vi "FCI Lip gap.vi"(8 "error in (no error)":errorcluster, 11 "Image 2":T1) -> (0 "error IO":errorcluster, 2 "Lip Gap":sgl format="%.2f")   [LabVIEW 2019, in "Algorithm.lvclass"]
uses:
  FrameworkOverrides/Algorithm.lvclass
  <vilib>/vision/NI_Vision_Development_Module.lvlib
  <vilib>/vision/Measure.llb/Straight Edge Process.ctl
  <vilib>/vision/Measure.llb/Straight Edge Options.ctl
  <vilib>/vision/Measure.llb/Edge Polarity.ctl
  <vilib>/vision/Measure.llb/Edge Options.ctl
  <vilib>/vision/Image Controls.llb/IMAQ Image.ctl
panel:
  out "Image":T1(plugin-control)
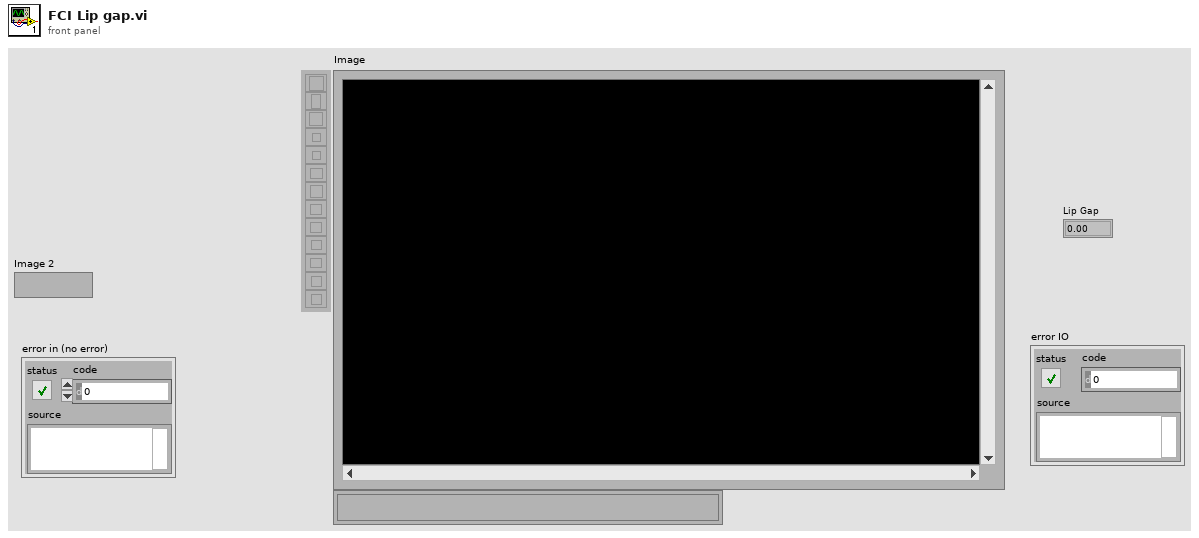
[diagram p1: front panel]
types:
  T1 = typedef "IMAQ Image.ctl" = refnum<image>
  T2 = cluster{"Left":dbl, "Top":dbl, "Right":dbl, "Bottom":dbl, "Angle":dbl}
  T3 = typedef "Edge Options.ctl" = cluster{"Edge Polarity":T4, "Kernel Size":u32, "Width":u32, "Minimum Edge Strength":sgl, "Interpolation Type":enum32{"Zero Order", "Bilinear", "Quadratic", "Cubic", "Bilinear Fixed"}, "Data Processing Method":enum32{"Average", "Median"}}
  T4 = typedef "Edge Polarity.ctl" = u32
  T5 = enum16{"Get First Edge", "Get First + Last Edge", "Get All Edges", "Get Best Edge"}
  T6 = cluster{"Search Direction":u32, "Edge Options":T3, "Show Search Area":bool, "Show Search Lines":bool, "Show Edges Found":bool, "Show Result":bool, "Search Area Color":u32, "Search Lines Color":u32, "Edge Locations Color":u32, "Result Color":u32, "Overlay Group Name":string}
  T7 = typedef "Straight Edge Options.ctl" = cluster{"Number of Lines":i32, "Type":T8, "Min. Score":dbl, "Max. Score":dbl, "Orientation":dbl, "Angle Range":dbl, "Angle Tolerance":dbl, "Step Size":u32, "Min. SNR (db)":dbl, "Min. Points (%)":dbl, "Hough Iterations":i32}
  T8 = typedef "Straight Edge Process.ctl" = enum32{"First Edge Rake", "Best Edge Rake", "Hough Edge Rake", "First Edge Projection", "Best Edge Projection"}
  T9 = typedef "Image Type" = u32
  T10 = typedef "ROI Descriptor" = cluster{"Global Rectangle":i32[], "Contours":cluster{"ID":enum32{"External", "Internal"}, "Type":u32, "Coordinates":i32[]}[]}
  T11 = cluster{"Point1 (Pixels)":cluster{"X":sgl, "Y":sgl}, "Point2 (Pixels)":cluster{"X":sgl, "Y":sgl}, "Point1 (Real-World)":cluster{"X":sgl, "Y":sgl}, "Point2 (Real-World)":cluster{"X":sgl, "Y":sgl}, "Angle (Pixel)":dbl, "Angle (Real-World)":dbl, "Score":dbl, "Straightness":dbl, "Average SNR (db)":dbl, "Calibration Valid":bool}[]
  T12 = cluster{"Point1 (Pixels)":cluster{"X":sgl, "Y":sgl}, "Point2 (Pixels)":cluster{"X":sgl, "Y":sgl}, "Point1 (Real-World)":cluster{"X":sgl, "Y":sgl}, "Point2 (Real-World)":cluster{"X":sgl, "Y":sgl}, "Angle (Pixel)":dbl, "Angle (Real-World)":dbl, "Score":dbl, "Straightness":dbl, "Average SNR (db)":dbl, "Calibration Valid":bool}
  T13 = typedef "Edge New.ctl" = cluster{"Location (Pixel)":cluster{"X":sgl, "Y":sgl}, "Location (Real-World)":cluster{"X":sgl, "Y":sgl}, "Distance (Pixel)":dbl, "Distance (Real-World)":dbl, "Strength":dbl, "Noise":dbl, "Rising?":bool}
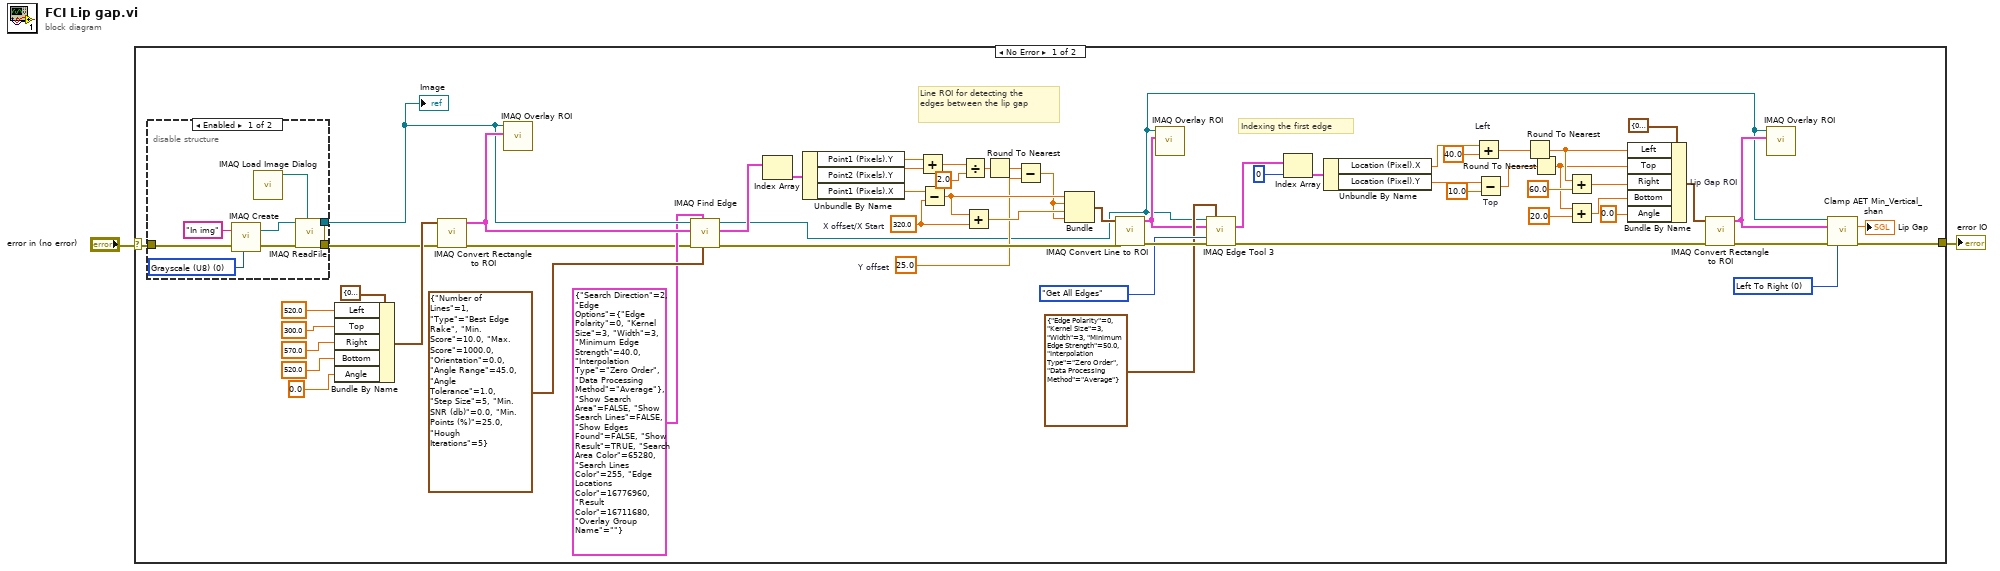
[diagram p0: block diagram]
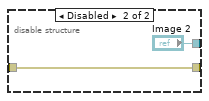
[diagram p2: hidden frame]
diagram:
  n1 = case shown="No Error" "error in (no error)" {
    selector: "error in (no error)" -> [w61 w72]
    tunnel: [w3 w72] -> w1
    frame No Error {
      w6 = u16 0 items=["Left To Right", "Right To Left", "Top To Bottom", "Bottom To Top"] ("Scanning axis")
      w29 = sgl 25.0  # Y offset
      w38 = sgl 320.0  # X offset/X Start
      # "Indexing the first edge"
      # "Line ROI for detecting the edges between the lip gap"
      n2 = disable-structure shown="Enabled" {
        disable-tunnel: w61 -> [w64 w71]
        disable-tunnel: [w63 w71] -> w58
        disable-tunnel: [w62 "Image 2"] -> w51
        frame Enabled {
          w67 = T9 0 items=["Grayscale (U8)", "Grayscale (I16)", "Grayscale (SGL)", "Complex (CSG)", "RGB (U32)", "HSL (U32)", "RGB (U64)", "Grayscale (U16)"] ("Image Type")
          n3 = call "IMAQ Create"("Image Name"="In img", "Image Type"=w67, "error in (no error)"=w64) -> ("New Image"=w69:T1, "error out"=w66:errorcluster)  [unwired: 2 in]
          n4 = call "IMAQ Load Image Dialog"() -> ("Path"=w65:path)  [unwired: 9 in, 2 out]
          n5 = call "IMAQ ReadFile"("File Path"=w65, "error in (no error)"=w66, "Image"=w69) -> ("error out"=w63:errorcluster, "Image Out"=w62:T1)  [unwired: 4 in, 3 out]
        }
        frame Disabled {
        }
      }
      "Image" <- w51
      n6 = Bundle By Name(cluster=T2 {"Left"=0.0, "Top"=0.0, "Right"=0.0, "Bottom"=0.0, "Angle"=0.0} ("input cluster"), "Left"=520.0, "Top"=300.0, "Right"=570.0, "Bottom"=520.0, "Angle"=0.0) -> (w59:T2)
      n7 = call "IMAQ Convert Rectangle to ROI"("error in (no error)"=w58, "Rectangle"=w59) -> ("error out"=w4:errorcluster, "ROI Descriptor"=w52:T10)  [unwired: 7 in]
      n8 = call "IMAQ Overlay ROI"("ROI Descriptor"=w52, "Image"=w51) -> ()  [unwired: 8 in, 2 out]
      n9 = call "IMAQ Find Edge"("Line Fit Options"=T7 {"Number of Lines"=1, "Type"=enum."Best Edge Rake", "Min. Score"=10.0, "Max. Score"=1000.0, "Orientation"=0.0, "Angle Range"=45.0, "Angle Tolerance"=1.0, "Step Size"=5, "Min. SNR (db)"=0.0, "Min. Points (%)"=25.0, "Hough Iterations"=5}, "Options"=T6 {"Search Direction"=2, "Edge Options"={"Edge Polarity"=0, "Kernel Size"=3, "Width"=3, "Minimum Edge Strength"=40.0, "Interpolation Type"=enum."Zero Order", "Data Processing Method"=enum."Average"}, "Show Search Area"=FALSE, "Show Search Lines"=FALSE, "Show Edges Found"=FALSE, "Show Result"=TRUE, "Search Area Color"=65280, "Search Lines Color"=255, "Edge Locations Color"=16776960, "Result Color"=16711680, "Overlay Group Name"=""}, "error in (no error)"=w4, "ROI Descriptor"=w52, "Image"=w51) -> ("error out"=w36:errorcluster, "Straight Edges"=w48:T11, "Image Out"=w7:T1)  [unwired: 3 in, 1 out]
      n10 = Index Array(array=w48) -> (element=w47:T12)  [unwired: 1 in]
      n11 = Unbundle By Name(w47) -> ("Point1 (Pixels).Y"=w46:sgl, "Point2 (Pixels).Y"=w45:sgl, "Point1 (Pixels).X"=w41:sgl)
      n12 = Add(x=w46, y=w45) -> (x+y=w44:sgl)
      n13 = Subtract(x=w41, y=w38) -> (x-y=w40:sgl)
      n14 = Divide(x=w44, y=sgl 2.0) -> (x/y=w42:sgl)
      n15 = Add(x=w40, y=w38) -> (x+y=w39:sgl)
      n16 = Round To Nearest(number=w42) -> (nearest integer value=w30:sgl)
      n17 = Subtract(x=w30, y=w29) -> (x-y=w31:sgl)
      n18 = Bundle(w40, w31, w39, w31) -> (w37:cluster{sgl, sgl, sgl, sgl})  [unwired: 1 in]
      n19 = call "IMAQ Convert Line to ROI"("error in (no error)"=w36, "Line"=w37) -> ("error out"=w35:errorcluster, "ROI Descriptor"=w32:T10)  [unwired: 7 in]
      n20 = call "IMAQ Overlay ROI"("ROI Descriptor"=w32, "Image"=w7) -> ()  [unwired: 8 in, 2 out]
      n21 = call "IMAQ Edge Tool 3"("Image"=w7, "Edge Options"=T3 {"Edge Polarity"=0, "Kernel Size"=3, "Width"=3, "Minimum Edge Strength"=50.0, "Interpolation Type"=enum."Zero Order", "Data Processing Method"=enum."Average"}, "ROI Descriptor"=w32, "Process"=T5."Get All Edges", "error in (no error)"=w35) -> ("Edge Information"=w28:T13[], "error out"=w16:errorcluster)  [unwired: 6 in, 3 out]
      n22 = Index Array(array=w28, index=0) -> (element=w27:T13)
      n23 = Unbundle By Name(w27) -> ("Location (Pixel).X"=w23:sgl, "Location (Pixel).Y"=w21:sgl)
      n24 = Add "Left"(x=w23, y=sgl 40.0) -> (x+y=w19:sgl)
      n25 = Subtract "Top"(x=w21, y=sgl 10.0) -> (x-y=w18:sgl)
      n26 = Round To Nearest(number=w19) -> (nearest integer value=w15:sgl)
      n27 = Round To Nearest(number=w18) -> (nearest integer value=w11:sgl)
      n28 = Add(x=w15, y=60.0 ("Right")) -> (x+y=w13:dbl)
      n29 = Add(x=w11, y=20.0 ("Bottom")) -> (x+y=w10:dbl)
      n30 = Bundle By Name "Lip Gap ROI"(cluster=T2 {"Left"=0.0, "Top"=0.0, "Right"=0.0, "Bottom"=0.0, "Angle"=0.0} ("input cluster"), "Left"=w15, "Top"=w11, "Right"=w13, "Bottom"=w10, "Angle"=0.0) -> (w17:T2)
      n31 = call "IMAQ Convert Rectangle to ROI"("error in (no error)"=w16, "Rectangle"=w17) -> ("error out"=w9:errorcluster, "ROI Descriptor"=w8:T10)  [unwired: 7 in]
      n32 = call "IMAQ Overlay ROI"("ROI Descriptor"=w8, "Image"=w7) -> ()  [unwired: 8 in, 2 out]
      n33 = call "Clamp AET Min_Vertical_shan.vi"("Image"=w7, "Scanning axis"=w6, "ROI Descriptor"=w8, "error in (no error)"=w9) -> ("Distance"=→"Lip Gap":sgl, "error out"=w3:errorcluster)  [unwired: 5 in, 5 out]
    }
    frame Error {
    }
  }
  "error IO" <- w1
